vi "LSMcontroller_v56_from here for labview64bit.vi"() -> ()   [LabVIEW 2015] (continued)
                                tunnel: w3219 -> [_ w3224]
                                frame False {
                                }
                                frame True {
                                n918 = Quotient & Remainder(x=w3224, y=u32 2 ("min phot")) -> (floor(x/y)=w3223:u32)  [unwired: 1 out]
                                n919 = Max & Min(x=w3223, y=u32 5) -> (max(x,y)=w3222:u32)  [unwired: 1 out]
                                n920 = local write "min phot"(w3222) -> ()
                                }
                                }
                                n921 = To Double Precision Float(number=w3209) -> (double precision float=w3210:dbl)
                                n922 = local write "img_CH1"(w3211) -> ()
                                n923 = property on="img_CH1" class="IntGraph (strict)"("ZScale.Maximum"=w3210) -> ()  [unwired: 2 in, 2 out]
                                }
                                }
                                }
                                frame #4 {
                                w3228 = u16 1 items=["Stream to disk", "Post process", "real time process"] ("Ring")
                                n924 = local read "T3R Data processing"() -> (w3227:u16)
                                n925 = Equal?(x=w3227, y=w3228) -> (x = y?=w3226:bool)
                                n926 = case shown="False" w3226 {
                                frame False {
                                # "intensity"
                                n927 = local read "Current Average"() -> (w3233:sgl)
                                n928 = local read "image2list"() -> (w3229:u16)
                                n929 = local read "image1list"() -> (w3230:u16)
                                n930 = call "dattoimage.vi"("image2list"=w3229, "Current Average"=w3233, "image1list"=w3230) -> ("image 1 array out"=w3232:sgl[][])  [unwired: 1 out]
                                n931 = Transpose 2D Array(2D array=w3232) -> (transposed array=w3231:sgl[][])
                                n932 = local write "img_CH2"(w3231) -> ()
                                }
                                frame True {
                                }
                                }
                                }
                                }
                              }
                              frame Enabled {
                              }
                            }
                          }
                        }
                        n933 = local write "64bit disabled"(TRUE ("64bit disabled")) -> ()
                      }
                      frame #9 {
                        n934 = call "2pparameters.vi"("command"="get") -> ("params out"=w3236:T12)  [unwired: 1 in]
                        n935 = Unbundle By Name(w3236) -> ("auto OD"=w3235:bool)
                        n936 = case shown="True" w3235 {
                          frame False {
                          }
                          frame True {
                            n937 = call "configuration.vi"("command"="get") -> ("config out"=w3239:T13)  [unwired: 2 in, 1 out]
                            n938 = call "2pparameters.vi"("command"="get") -> ("params out"=w3242:T12)  [unwired: 1 in]
                            n939 = Unbundle By Name(w3239) -> ("image OD"=w3237:u16)
                            n940 = Unbundle By Name(w3242) -> ("ODfilt"=w3238:u16)
                            n941 = call "filterwheelcontrol_nothorlabslib.vi"("Current OD filt"=w3237, "New ODfilt"=w3238) -> ()  [unwired: 1 in]
                          }
                        }
                        n942 = call "reset AO_DO_v3.vi"() -> ()  [unwired: 12 in]
                      }
                      frame #10 {
                        n943 = stacked-sequence {
                          tunnel: w3256 -> [w3259 _ _ _ _ _]
                          tunnel: w3255 -> [w3258 _ _ _ _ _]
                          tunnel: w3254 -> [w3257 _ _ _ _ _]
                          tunnel: w3253 -> [_ w3308 _ _ _ _]
                          tunnel: w3252 -> [_ w3307 w3362 w3459 _ _]
                          tunnel: w3251 -> [_ w3306 w3361 w3458 _ _]
                          tunnel: w3250 -> [_ _ w3360 _ _ _]
                          tunnel: w3249 -> [_ _ w3359 _ _ _]
                          tunnel: w3248 -> [_ _ _ w3457 _ _]
                          tunnel: w3247 -> [_ _ _ w3456 _ _]
                          tunnel: w3246 -> [_ _ w3357 _ _ _]
                          tunnel: w3245 -> [_ _ w3356 _ _ _]
                          tunnel: w3244 -> [_ _ _ w3454 _ _]
                          tunnel: w3243 -> [_ _ _ w3453 _ _]
                          frame #0 {
                            n944 = case shown="False" w3259 {
                              tunnel: w3258 -> [_ w3281]
                              tunnel: w3257 -> [_ w3280]
                              frame True {
                                n945 = stacked-sequence {
                                seq-local: [w3260 _ _] -> [_ w3272 w3277]
                                frame #0 {
                                n946 = call "configuration.vi"("command"="get") -> ("config out"=w3266:T13)  [unwired: 2 in, 1 out]
                                n947 = Unbundle By Name(w3266) -> ("Voltage to Xgalvo"=w3263:i32)
                                n948 = call "2pparameters.vi"("command"="get") -> ("params out"=w3264:T12)  [unwired: 1 in]
                                n949 = in-place {
                                in-place-border: w3263 -> [w3271]
                                in-place-border: [w3268] -> w3260
                                n950 = in-place-cluster #9(w3264) -> ("aAO"=w3270:u32[])
                                n951 = call "remove channel from active arrayv2.vi"("line array in"=w3270, "line to remove"=w3271) -> ("line array out"=w3269:u32[], "index"=w3268:i32)  [unwired: 1 out]
                                n952 = in-place-cluster #9("aAO"=w3269) -> (w3261:T12)
                                }
                                n953 = call "2pparameters.vi"("Params in"=w3261, "command"="set") -> ()  [unwired: 1 out]
                                }
                                frame #1 {
                                n954 = call "waveformparamsv2.vi"("command"="rem AO", "index"=w3272) -> ()  [unwired: 3 in, 3 out]
                                }
                                frame #2 {
                                n955 = call "waveformsAObuffer.vi"("command"="get") -> ("AO wf out"=w3278:waveform(dbl)[])  [unwired: 1 in]
                                n956 = Delete From Array(array=w3278, length=1, index=w3277) -> (array with subset deleted=w3274:waveform(dbl)[])  [unwired: 1 out]
                                n957 = call "waveformsAObuffer.vi"("AO wf in"=w3274, "command"="set") -> ()  [unwired: 1 out]
                                }
                                }
                              }
                              frame False {
                                n958 = stacked-sequence {
                                seq-local: [w3282 _ _] -> [_ w3290 w3301]
                                tunnel: w3281 -> [_ w3289 _]
                                tunnel: w3280 -> [_ _ w3300]
                                frame #0 {
                                n959 = call "configuration.vi"("command"="get") -> ("config out"=w3287:T13)  [unwired: 2 in, 1 out]
                                n960 = Unbundle By Name(w3287) -> ("Voltage to Xgalvo"=w3283:i32)
                                n961 = call "2pparameters.vi"("command"="get") -> ("params out"=w3286:T12)  [unwired: 1 in]
                                n962 = Unbundle By Name(w3286) -> ("aAO"=w3284:u32[])
                                n963 = Search 1D Array(1D array=w3284, element=w3283) -> (index of element=w3282:i32)  [unwired: 1 in]
                                }
                                frame #1 {
                                n964 = call "waveformparamsv2.vi"("command"="get") -> ("Params out"=w3293:T16)  [unwired: 4 in, 2 out]
                                n965 = in-place {
                                in-place-border: w3290 -> [w3297]
                                in-place-border: w3289 -> [w3296]
                                n966 = in-place-cluster #10(w3293) -> ("AO parameters"=w3298:T17)
                                n967 = in-place {
                                in-place-border: w3296 -> [w3299]
                                n968 = in-place-array #11(w3298, w3297) -> ()  [unwired: 1 out]
                                n969 = in-place-array #11(w3299) -> (w3295:T17)  [unwired: 1 out]
                                }
                                n970 = in-place-cluster #10("AO parameters"=w3295) -> (w3291:T16)
                                }
                                n971 = call "waveformparamsv2.vi"("command"="set", "Params in"=w3291) -> ()  [unwired: 3 in, 3 out]
                                }
                                frame #2 {
                                n972 = call "waveformsAObuffer.vi"("command"="get") -> ("AO wf out"=w3304:waveform(dbl)[])  [unwired: 1 in]
                                n973 = Replace Array Subset(array=w3304, new element=w3300, index=w3301) -> (w3302:waveform(dbl)[])
                                n974 = call "waveformsAObuffer.vi"("AO wf in"=w3302, "command"="set") -> ()  [unwired: 1 out]
                                }
                                }
                              }
                            }
                          }
                          frame #1 {
                            n975 = case shown="True" w3308 {
                              tunnel: w3307 -> [_ w3330]
                              tunnel: w3306 -> [_ w3329]
                              frame True {
                                n976 = stacked-sequence {
                                seq-local: [w3309 _ _] -> [_ w3321 w3326]
                                frame #0 {
                                n977 = call "configuration.vi"("command"="get") -> ("config out"=w3315:T13)  [unwired: 2 in, 1 out]
                                n978 = Unbundle By Name(w3315) -> ("Voltage to Ygalvo"=w3312:i32)
                                n979 = call "2pparameters.vi"("command"="get") -> ("params out"=w3313:T12)  [unwired: 1 in]
                                n980 = in-place {
                                in-place-border: w3312 -> [w3320]
                                in-place-border: [w3317] -> w3309
                                n981 = in-place-cluster #12(w3313) -> ("aAO"=w3319:u32[])
                                n982 = call "remove channel from active arrayv2.vi"("line array in"=w3319, "line to remove"=w3320) -> ("line array out"=w3318:u32[], "index"=w3317:i32)  [unwired: 1 out]
                                n983 = in-place-cluster #12("aAO"=w3318) -> (w3310:T12)
                                }
                                n984 = call "2pparameters.vi"("Params in"=w3310, "command"="set") -> ()  [unwired: 1 out]
                                }
                                frame #1 {
                                n985 = call "waveformparamsv2.vi"("command"="rem AO", "index"=w3321) -> ()  [unwired: 3 in, 3 out]
                                }
                                frame #2 {
                                n986 = call "waveformsAObuffer.vi"("command"="get") -> ("AO wf out"=w3327:waveform(dbl)[])  [unwired: 1 in]
                                n987 = Delete From Array(array=w3327, length=1, index=w3326) -> (array with subset deleted=w3323:waveform(dbl)[])  [unwired: 1 out]
                                n988 = call "waveformsAObuffer.vi"("AO wf in"=w3323, "command"="set") -> ()  [unwired: 1 out]
                                }
                                }
                              }
                              frame False {
                                n989 = stacked-sequence {
                                seq-local: [w3331 _ _] -> [_ w3339 w3350]
                                tunnel: w3330 -> [_ w3338 _]
                                tunnel: w3329 -> [_ _ w3349]
                                frame #0 {
                                n990 = call "configuration.vi"("command"="get") -> ("config out"=w3336:T13)  [unwired: 2 in, 1 out]
                                n991 = Unbundle By Name(w3336) -> ("Voltage to Ygalvo"=w3332:i32)
                                n992 = call "2pparameters.vi"("command"="get") -> ("params out"=w3335:T12)  [unwired: 1 in]
                                n993 = Unbundle By Name(w3335) -> ("aAO"=w3333:u32[])
                                n994 = Search 1D Array(1D array=w3333, element=w3332) -> (index of element=w3331:i32)  [unwired: 1 in]
                                }
                                frame #1 {
                                n995 = call "waveformparamsv2.vi"("command"="get") -> ("Params out"=w3342:T16)  [unwired: 4 in, 2 out]
                                n996 = in-place {
                                in-place-border: w3339 -> [w3346]
                                in-place-border: w3338 -> [w3345]
                                n997 = in-place-cluster #13(w3342) -> ("AO parameters"=w3347:T17)
                                n998 = in-place {
                                in-place-border: w3345 -> [w3348]
                                n999 = in-place-array #14(w3347, w3346) -> ()  [unwired: 1 out]
                                n1000 = in-place-array #14(w3348) -> (w3344:T17)  [unwired: 1 out]
                                }
                                n1001 = in-place-cluster #13("AO parameters"=w3344) -> (w3340:T16)
                                }
                                n1002 = call "waveformparamsv2.vi"("command"="set", "Params in"=w3340) -> ()  [unwired: 3 in, 3 out]
                                }
                                frame #2 {
                                n1003 = call "waveformsAObuffer.vi"("command"="get") -> ("AO wf out"=w3353:waveform(dbl)[])  [unwired: 1 in]
                                n1004 = Replace Array Subset(array=w3353, new element=w3349, index=w3350) -> (w3351:waveform(dbl)[])
                                n1005 = call "waveformsAObuffer.vi"("AO wf in"=w3351, "command"="set") -> ()  [unwired: 1 out]
                                }
                                }
                              }
                            }
                          }
                          frame #2 {
                            n1006 = Build Array(w3357, w3356) -> (w3355:bool[])
                            n1007 = Boolean Array To Number(Boolean array=w3355) -> (number=w3358:u32)
                            n1008 = case shown="0" w3358 {
                              tunnel: w3362 -> [_ _ w3405]
                              tunnel: w3361 -> [_ _ w3404]
                              tunnel: w3360 -> [_ w3384 w3402]
                              tunnel: w3359 -> [_ w3383 w3403]
                              frame 1, Default {
                                n1009 = stacked-sequence {
                                seq-local: [w3363 _ _] -> [_ w3375 w3380]
                                frame #0 {
                                n1010 = call "configuration.vi"("command"="get") -> ("config out"=w3369:T13)  [unwired: 2 in, 1 out]
                                n1011 = Unbundle By Name(w3369) -> ("2P shutter"=w3366:i32)
                                n1012 = call "2pparameters.vi"("command"="get") -> ("params out"=w3367:T12)  [unwired: 1 in]
                                n1013 = in-place {
                                in-place-border: w3366 -> [w3374]
                                in-place-border: [w3371] -> w3363
                                n1014 = in-place-cluster #15(w3367) -> ("aDO"=w3373:u32[])
                                n1015 = call "remove channel from active arrayv2.vi"("line array in"=w3373, "line to remove"=w3374) -> ("line array out"=w3372:u32[], "index"=w3371:i32)  [unwired: 1 out]
                                n1016 = in-place-cluster #15("aDO"=w3372) -> (w3364:T12)
                                }
                                n1017 = call "2pparameters.vi"("Params in"=w3364, "command"="set") -> ()  [unwired: 1 out]
                                }
                                frame #1 {
                                n1018 = call "waveformparamsv2.vi"("command"="rem DO", "index"=w3375) -> ()  [unwired: 3 in, 3 out]
                                }
                                frame #2 {
                                n1019 = call "waveformsDObuffer.vi"("command"="get") -> ("DO wf out"=w3381:digitalwaveform[])  [unwired: 1 in]
                                n1020 = Delete From Array(array=w3381, length=1, index=w3380) -> (array with subset deleted=w3377:digitalwaveform[])  [unwired: 1 out]
                                n1021 = call "waveformsDObuffer.vi"("DO wf in"=w3377, "command"="set") -> ()  [unwired: 1 out]
                                }
                                }
                              }
                              frame 2 {
                                n1022 = stacked-sequence {
                                tunnel: w3384 -> [_ w3395 _]
                                tunnel: w3383 -> [_ _ w3399]
                                frame #0 {
                                n1023 = call "configuration.vi"("command"="get") -> ("config out"=w3386:T13)  [unwired: 2 in, 1 out]
                                n1024 = call "2pparameters.vi"("command"="get") -> ("params out"=w3390:T12)  [unwired: 1 in]
                                n1025 = Unbundle By Name(w3386) -> ("2P shutter"=w3385:i32)
                                n1026 = in-place {
                                in-place-border: w3385 -> [w3394]
                                n1027 = in-place-cluster #16(w3390) -> ("aDO"=w3393:u32[])
                                n1028 = call "add channel to active arrayv2.vi"("line array in"=w3393, "line to add"=w3394) -> ("line array out"=w3392:u32[])  [unwired: 2 out]
                                n1029 = in-place-cluster #16("aDO"=w3392) -> (w3388:T12)
                                }
                                n1030 = call "2pparameters.vi"("Params in"=w3388, "command"="set") -> ()  [unwired: 1 out]
                                }
                                frame #1 {
                                n1031 = call "waveformparamsv2.vi"("command"="add DO", "add DO"=w3395) -> ()  [unwired: 3 in, 3 out]
                                }
                                frame #2 {
                                n1032 = call "waveformsDObuffer.vi"("command"="get") -> ("DO wf out"=w3400:digitalwaveform[])  [unwired: 1 in]
                                n1033 = Build Array (concatenate)(w3400, w3399) -> (w3398:digitalwaveform[])
                                n1034 = call "waveformsDObuffer.vi"("DO wf in"=w3398, "command"="set") -> ()  [unwired: 1 out]
                                }
                                }
                              }
                              frame 0 {
                                n1035 = stacked-sequence {
                                seq-local: [w3406 _ _] -> [_ w3414 w3436]
                                tunnel: w3405 -> [_ _ _]
                                tunnel: w3404 -> [_ _ _]
                                tunnel: w3403 -> [_ _ w3435]
                                tunnel: w3402 -> [_ w3413 _]
                                frame #0 {
                                n1036 = call "configuration.vi"("command"="get") -> ("config out"=w3411:T13)  [unwired: 2 in, 1 out]
                                n1037 = call "2pparameters.vi"("command"="get") -> ("params out"=w3410:T12)  [unwired: 1 in]
                                n1038 = Unbundle By Name(w3411) -> ("2P shutter"=w3407:i32)
                                n1039 = Unbundle By Name(w3410) -> ("aDO"=w3408:u32[])
                                n1040 = Search 1D Array(1D array=w3408, element=w3407) -> (index of element=w3406:i32)  [unwired: 1 in]
                                }
                                frame #1 {
                                n1041 = call "2pparameters.vi"("command"="get") -> ("params out"=w3417:T12)  [unwired: 1 in]
                                n1042 = Unbundle By Name(w3417) -> ("wavdet"=w3415:bool, "autoshutter"=w3416:bool)
                                n1043 = case shown="True" w3416 {
                                tunnel: w3414 -> [_ w3421]
                                tunnel: w3415 -> [_ w3420]
                                tunnel: w3413 -> [_ w3419]
                                frame False {
                                }
                                frame True {
                                n1044 = case shown="False" w3420 {
                                tunnel: w3421 -> [w3425 _]
                                tunnel: w3419 -> [w3423 _]
                                frame False {
                                n1045 = Index Array(array=w3423, index=0) -> (element=w3422:T20)
                                n1046 = call "waveformparamsv2.vi"("command"="get") -> ("Params out"=w3428:T16)  [unwired: 4 in, 2 out]
                                n1047 = in-place {
                                in-place-border: w3425 -> [w3432]
                                in-place-border: w3422 -> [w3430]
                                n1048 = in-place-cluster #17(w3428) -> ("DO parameters"=w3433:T19)
                                n1049 = in-place {
                                in-place-border: w3430 -> [w3434]
                                n1050 = in-place-array #18(w3433, w3432) -> ()  [unwired: 1 out]
                                n1051 = in-place-array #18(w3434) -> (w3431:T19)  [unwired: 1 out]
                                }
                                n1052 = in-place-cluster #17("DO parameters"=w3431) -> (w3426:T16)
                                }
                                n1053 = call "waveformparamsv2.vi"("command"="set", "Params in"=w3426) -> ()  [unwired: 3 in, 3 out]
                                }
                                frame True {
                                }
                                }
                                }
                                }
                                }
                                frame #2 {
                                n1054 = call "2pparameters.vi"("command"="get") -> ("params out"=w3439:T12)  [unwired: 1 in]
                                n1055 = Unbundle By Name(w3439) -> ("wavdet"=w3437:bool, "autoshutter"=w3438:bool)
                                n1056 = case shown="True" w3438 {
                                tunnel: w3436 -> [_ w3443]
                                tunnel: w3437 -> [_ w3442]
                                tunnel: w3435 -> [_ w3441]
                                frame False {
                                }
                                frame True {
                                n1057 = case shown="False" w3442 {
                                tunnel: w3443 -> [w3447 _]
                                tunnel: w3441 -> [w3446 _]
                                frame False {
                                n1058 = Index Array(array=w3446, index=0) -> (element=w3444:digitalwaveform)
                                n1059 = call "waveformsDObuffer.vi"("command"="get") -> ("DO wf out"=w3449:digitalwaveform[])  [unwired: 1 in]
                                n1060 = Replace Array Subset(array=w3449, new element=w3444, index=w3447) -> (w3451:digitalwaveform[])
                                n1061 = call "waveformsDObuffer.vi"("DO wf in"=w3451, "command"="set") -> ()  [unwired: 1 out]
                                }
                                frame True {
                                }
                                }
                                }
                                }
                                }
                                }
                              }
                            }
                          }
                          frame #3 {
                            n1062 = Build Array(w3454, w3453) -> (w3455:bool[])
                            n1063 = Boolean Array To Number(Boolean array=w3455) -> (number=w3452:u32)
                            n1064 = case shown="0" w3452 {
                              tunnel: w3459 -> [_ _ w3502]
                              tunnel: w3458 -> [_ _ w3501]
                              tunnel: w3457 -> [_ w3481 w3499]
                              tunnel: w3456 -> [_ w3480 w3500]
                              frame 1, Default {
                                n1065 = stacked-sequence {
                                seq-local: [w3460 _ _] -> [_ w3472 w3477]
                                frame #0 {
                                n1066 = call "configuration.vi"("command"="get") -> ("config out"=w3466:T13)  [unwired: 2 in, 1 out]
                                n1067 = Unbundle By Name(w3466) -> ("LT timestamp"=w3463:u32)
                                n1068 = call "2pparameters.vi"("command"="get") -> ("params out"=w3464:T12)  [unwired: 1 in]
                                n1069 = in-place {
                                in-place-border: w3463 -> [w3471]
                                in-place-border: [w3468] -> w3460
                                n1070 = in-place-cluster #19(w3464) -> ("aDO"=w3470:u32[])
                                n1071 = call "remove channel from active arrayv2.vi"("line array in"=w3470, "line to remove"=w3471) -> ("line array out"=w3469:u32[], "index"=w3468:i32)  [unwired: 1 out]
                                n1072 = in-place-cluster #19("aDO"=w3469) -> (w3461:T12)
                                }
                                n1073 = call "2pparameters.vi"("Params in"=w3461, "command"="set") -> ()  [unwired: 1 out]
                                }
                                frame #1 {
                                n1074 = call "waveformparamsv2.vi"("command"="rem DO", "index"=w3472) -> ()  [unwired: 3 in, 3 out]
                                }
                                frame #2 {
                                n1075 = call "waveformsDObuffer.vi"("command"="get") -> ("DO wf out"=w3478:digitalwaveform[])  [unwired: 1 in]
                                n1076 = Delete From Array(array=w3478, length=1, index=w3477) -> (array with subset deleted=w3474:digitalwaveform[])  [unwired: 1 out]
                                n1077 = call "waveformsDObuffer.vi"("DO wf in"=w3474, "command"="set") -> ()  [unwired: 1 out]
                                }
                                }
                              }
                              frame 2 {
                                n1078 = stacked-sequence {
                                tunnel: w3481 -> [_ _ w3494]
                                tunnel: w3480 -> [_ w3492 _]
                                frame #0 {
                                n1079 = call "configuration.vi"("command"="get") -> ("config out"=w3483:T13)  [unwired: 2 in, 1 out]
                                n1080 = Unbundle By Name(w3483) -> ("LT timestamp"=w3482:u32)
                                n1081 = call "2pparameters.vi"("command"="get") -> ("params out"=w3487:T12)  [unwired: 1 in]
                                n1082 = in-place {
                                in-place-border: w3482 -> [w3491]
                                n1083 = in-place-cluster #20(w3487) -> ("aDO"=w3490:u32[])
                                n1084 = call "add channel to active arrayv2.vi"("line array in"=w3490, "line to add"=w3491) -> ("line array out"=w3489:u32[])  [unwired: 2 out]
                                n1085 = in-place-cluster #20("aDO"=w3489) -> (w3485:T12)
                                }
                                n1086 = call "2pparameters.vi"("Params in"=w3485, "command"="set") -> ()  [unwired: 1 out]
                                }
                                frame #1 {
                                n1087 = call "waveformparamsv2.vi"("command"="add DO", "add DO"=w3492) -> ()  [unwired: 3 in, 3 out]
                                }
                                frame #2 {
                                n1088 = call "waveformsDObuffer.vi"("command"="get") -> ("DO wf out"=w3497:digitalwaveform[])  [unwired: 1 in]
                                n1089 = Build Array (concatenate)(w3497, w3494) -> (w3496:digitalwaveform[])
                                n1090 = call "waveformsDObuffer.vi"("DO wf in"=w3496, "command"="set") -> ()  [unwired: 1 out]
                                }
                                }
                              }
                              frame 0 {
                                n1091 = stacked-sequence {
                                seq-local: [w3503 _ _] -> [_ w3513 w3530]
                                tunnel: w3502 -> [_ _ _]
                                tunnel: w3501 -> [_ _ _]
                                tunnel: w3500 -> [_ w3510 _]
                                tunnel: w3499 -> [_ _ w3529]
                                frame #0 {
                                n1092 = call "configuration.vi"("command"="get") -> ("config out"=w3508:T13)  [unwired: 2 in, 1 out]
                                n1093 = Unbundle By Name(w3508) -> ("LT timestamp"=w3504:u32)
                                n1094 = call "2pparameters.vi"("command"="get") -> ("params out"=w3507:T12)  [unwired: 1 in]
                                n1095 = Unbundle By Name(w3507) -> ("aDO"=w3505:u32[])
                                n1096 = Search 1D Array(1D array=w3505, element=w3504) -> (index of element=w3503:i32)  [unwired: 1 in]
                                }
                                frame #1 {
                                n1097 = local read "Measurement"() -> (w3512:T5)
                                n1098 = To Unsigned Long Integer(number=w3512) -> (unsigned 32bit integer=w3511:u32)
                                n1099 = case shown="5..7" w3511 {
                                tunnel: w3513 -> [_ w3517]
                                tunnel: w3510 -> [_ w3514]
                                frame 0..4, Default {
                                }
                                frame 5..7 {
                                n1100 = Index Array(array=w3514, index=0) -> (element=w3515:T20)
                                n1101 = call "waveformparamsv2.vi"("command"="get") -> ("Params out"=w3520:T16)  [unwired: 4 in, 2 out]
                                n1102 = in-place {
                                in-place-border: w3517 -> [w3524]
                                in-place-border: w3515 -> [w3522]
                                n1103 = in-place-cluster #21(w3520) -> ("DO parameters"=w3525:T19)
                                n1104 = in-place {
                                in-place-border: w3522 -> [w3526]
                                n1105 = in-place-array #22(w3525, w3524) -> ()  [unwired: 1 out]
                                n1106 = in-place-array #22(w3526) -> (w3523:T19)  [unwired: 1 out]
                                }
                                n1107 = in-place-cluster #21("DO parameters"=w3523) -> (w3518:T16)
                                }
                                n1108 = call "waveformparamsv2.vi"("command"="set", "Params in"=w3518) -> ()  [unwired: 3 in, 3 out]
                                }
                                }
                                }
                                frame #2 {
                                n1109 = local read "Measurement"() -> (w3528:T5)
                                n1110 = To Unsigned Long Integer(number=w3528) -> (unsigned 32bit integer=w3527:u32)
                                n1111 = case shown="5..7" w3527 {
                                tunnel: w3530 -> [_ w3534]
                                tunnel: w3529 -> [_ w3532]
                                frame 0..4, Default {
                                }
                                frame 5..7 {
                                n1112 = Index Array(array=w3532, index=0) -> (element=w3531:digitalwaveform)
                                n1113 = call "waveformsDObuffer.vi"("command"="get") -> ("DO wf out"=w3536:digitalwaveform[])  [unwired: 1 in]
                                n1114 = Replace Array Subset(array=w3536, new element=w3531, index=w3534) -> (w3538:digitalwaveform[])
                                n1115 = call "waveformsDObuffer.vi"("DO wf in"=w3538, "command"="set") -> ()  [unwired: 1 out]
                                }
                                }
                                }
                                }
                              }
                            }
                          }
                          frame #4 {
                            n1116 = call "Used AO lines.vi"() -> ("used AO names"=w3541:string[], "used AO lines"=w3539:tag[])  [unwired: 2 in]
                            n1117 = control-ref of="Analog Lines Plot"() -> (w3540:refnum<vi>)
                            n1118 = control-ref of="Digital Lines Plot"() -> (w3542:refnum<vi>)
                            n1119 = call "Used DO lines.vi"() -> ("used DO names"=w3543:string[], "used DO lines"=w3544:tag[])  [unwired: 2 in]
                            n1120 = local write "Analog Used Lines"(w3539) -> ()
                            n1121 = local write "Analog Used Names"(w3541) -> ()
                            n1122 = local write "Digital Used Lines"(w3544) -> ()
                            n1123 = local write "Digital Used Names"(w3543) -> ()
                            n1124 = call "prepDOWaveplot.vi"("DigitalGraph in"=w3542, "used DO names"=w3543) -> ()  [unwired: 1 in]
                            n1125 = call "prepAOWaveplot.vi"("WaveformGraph in"=w3540, "Analog Used Names"=w3541) -> ()  [unwired: 1 in]
                          }
                          frame #5 {
                            n1126 = local read "Meastab"() -> (w3559:enum32{"X-Y Image", "Linescan", "Timetrace"})
                            n1127 = property on="refwf" class="Ring (strict)"() -> ("RingText.Text"=w3556:string)  [unwired: 2 in, 2 out]
                            n1128 = case shown="\"Timetrace\"" w3559 {
                              tunnel: [w3561 w3562] -> w3560
                              frame "X-Y Image", Default {
                                n1129 = local read "Sampling rate"() -> (w3561:dbl)
                              }
                              frame "Timetrace" {
                                n1130 = local read "srateAODOtt"() -> (w3562:dbl)
                              }
                            }
                            n1131 = call "waveformsAObuffer.vi"("command"="get") -> ("AO wf out"=w3547:waveform(dbl)[])  [unwired: 1 in]
                            n1132 = local read "wavdet"() -> (w3557:bool)
                            n1133 = call "waveformsDObuffer.vi"("command"="get") -> ("DO wf out"=w3551:digitalwaveform[])  [unwired: 1 in]
                            n1134 = call "correctwaveformsizetemp.vi"("new sampling frequency (Hz)"=w3560, "start"=FALSE, "reference waveforms to"=w3556, "Analog waveforms in"=w3547, "stop"=TRUE, "Digital waveforms in"=w3551) -> ("analog wf out"=w3553:waveform(dbl)[], "Digital wf out"=w3555:digitalwaveform[], "measpoints"=w3558:i32)
                            n1135 = local write "Analog Lines Plot"(w3553) -> ()
                            n1136 = call "GetNumCamFramesv2.vi"("Digital Waveform Graph"=w3555) -> ("Numeric"=w3554:i32)  [unwired: 10 in]
                            n1137 = local write "Digital Lines Plot"(w3555) -> ()
                            n1138 = call "waveformsDObuffer.vi"("DO wf in"=w3555, "command"="set") -> ()  [unwired: 1 out]
                            n1139 = call "waveformsAObuffer.vi"("AO wf in"=w3553, "command"="set") -> ()  [unwired: 1 out]
                            n1140 = local write "Total Camera Frames"(w3554) -> ()
                            n1141 = case shown="True" w3557 {
                              tunnel: w3558 -> [_ w3563]
                              frame False {
                              }
                              frame True {
                                n1142 = local write "# of frames"(w3563) -> ()
                              }
                            }
                          }
                        }
                        n1143 = call "stoperaseCI.vi"() -> ()  [unwired: 12 in]
                        n1144 = call "stoperaseDO_img.vi"() -> ()  [unwired: 12 in]
                        n1145 = call "stoperaseAO_img.vi"() -> ()  [unwired: 12 in]
                        n1146 = call "stoperaseAI_img.vi"() -> ()  [unwired: 12 in]
                      }
                      frame #11 {
                        w3571 = FALSE ("Value (Signaling)")
                        n1147 = local read "save\ndata"() -> (w3564:bool)
                        n1148 = local read "save\ndata"() -> (w3565:bool)
                        n1149 = property on="Stop" class="Bool (strict)"("Visible"=FALSE, "DisabledEnum"=T8."Disabled" ("Disabled")) -> ()  [unwired: 2 in, 2 out]
                        n1150 = case shown="True" w3564 {
                          frame False {
                          }
                          frame True {
                            n1151 = call "closetiffs.vi"() -> ()  [unwired: 12 in]
                          }
                        }
                        n1152 = case shown="True" w3565 {
                          tunnel: w3566 -> [_ w3572]
                          frame False {
                          }
                          frame True {
                            n1153 = local read "filename prefix"() -> (w3574:string)
                            n1154 = local read "data dir"() -> (w3573:path)
                            n1155 = call "savetimestamps.vi"("timestamp"=w3572, "filename prefix in"=w3574, "data dir in"=w3573) -> ()  [unwired: 1 in]
                            n1156 = call "saveparams.vi"("filename prefix in"=w3574, "data dir in"=w3573) -> ()  [unwired: 2 in]
                          }
                        }
                        n1157 = property on="Start" class="Bool (strict)"("Visible"=TRUE, "DisabledEnum"=T8."Enabled" ("Disabled")) -> ()  [unwired: 2 in, 2 out]
                        n1158 = property on="Start" class="Bool (strict)"("Val(Sgnl)"=w3571) -> ()  [unwired: 2 in, 2 out]
                        n1159 = property on="Stop" class="Bool (strict)"("Val(Sgnl)"=w3571) -> ()  [unwired: 2 in, 2 out]
                      }
                      frame #12 {
                        w3578 = T23 2 items=["no dialog", "OK message", "continue or stop message", "OK message + warnings", "continue/stop + warnings"] ("type of dialog (OK msg:1)")
                        n1160 = call "displayerrors.vi"() -> ("error IO"=w3577:errorcluster)
                        n1161 = call <vilib>:"General Error Handler.vi"("type of dialog (OK msg:1)"=w3578, "error in (no error)"=w3577) -> ("error out"=w3576:errorcluster)  [unwired: 9 in, 4 out]
                        n1162 = call <vilib>:"Clear Errors.vi"("error in (no error)"=w3576) -> ("error out"=w3575:errorcluster)  [unwired: 5 in, 1 out]
                        n1163 = call "seterrors.vi"("error IO"=w3575) -> ()
                      }
                    }
                  }
                  frame "X-Y-Z-t movie" {
                    n1164 = call "2pparameters.vi"("command"="get") -> ("params out"=w3581:T12)  [unwired: 1 in]
                    n1165 = Bundle By Name(cluster=w3581, "type"="X-Y-Z-t movie") -> (w3579:T12)
                    n1166 = call "2pparameters.vi"("Params in"=w3579, "command"="set") -> ()  [unwired: 1 out]
                  }
                  frame "linescan" {
                    n1167 = call "2pparameters.vi"("command"="get") -> ("params out"=w3586:T12)  [unwired: 1 in]
                    n1168 = Bundle By Name(cluster=w3586, "type"="linescan") -> (w3588:T12)
                    n1169 = call "2pparameters.vi"("Params in"=w3588, "command"="set") -> ()  [unwired: 1 out]
                  }
                  frame "Timetrace", "Lifetime (contour)" {
                    n1170 = local read "ttt"() -> (w3589:T4)
                    n1171 = case shown="\"Resonant Ellipse\", \"freeform contour\"" w3589 {
                      frame "Point", Default {
                        n1172 = stacked-sequence {
                          seq-local: [w3590 _ _ _ _ _ _ _ _] -> [_ _ w3723 _ _ _ _ _ w3781]
                          frame #0 {
                            n1173 = Get Date/Time In Seconds() -> (seconds since 1Jan1904=w3591:timestamp)
                            n1174 = call "createdatafolder.vi"("timestamp in"=w3591) -> ("current data path"=w3592:path, "timestamp out"=w3590:timestamp)
                            n1175 = stacked-sequence {
                              frame #0 {
                                n1176 = call "2pparameters.vi"("command"="get") -> ("params out"=w3607:T12)  [unwired: 1 in]
                                n1177 = Bundle By Name(cluster=w3607, "type"="Timetrace") -> (w3605:T12)
                                n1178 = call "2pparameters.vi"("command"="get") -> ("params out"=w3596:T12)  [unwired: 1 in]
                                n1179 = local write "graphtab"(T6."timetrace" ("graphtab")) -> ()
                                n1180 = Unbundle By Name(w3596) -> ("Vx-min Img"=w3598:dbl, "VX-max Img"=w3597:dbl, "Vy-min Img"=w3600:dbl, "Vy-max Img"=w3599:dbl, "Angle Img"=w3601:dbl)
                                n1181 = property on="Stop" class="Bool (strict)"("Visible"=TRUE, "DisabledEnum"=T8."Enabled" ("Disabled")) -> ()  [unwired: 2 in, 2 out]
                                n1182 = property on="Start" class="Bool (strict)"("Visible"=FALSE, "DisabledEnum"=T8."Disabled and Grayed Out" ("Disabled")) -> ()  [unwired: 2 in, 2 out]
                                n1183 = local read "Vy-ref"() -> (w3603:dbl)
                                n1184 = local read "Vx-ref"() -> (w3602:dbl)
                                n1185 = call "2pparameters.vi"("Params in"=w3605, "command"="set") -> ()  [unwired: 1 out]
                                n1186 = script code="Xic=(ximax+ximin)./2;\nYic=(yimax+yimin)./2;\nx=x-Xic;\ny=y-Yic;\nxout=x.*cos(pi/180.*phi)+y.*sin(pi./180.*phi)+Xic;\nyout=-x.*sin(pi./180.*phi)+y.*cos(pi./180.*phi)+Yic;"("ximax"=w3597, "ximin"=w3598, "yimax"=w3599, "yimin"=w3600, "phi"=w3601, "x"=w3602, "y"=w3603) -> ("xout"=w3594:dbl, "yout"=w3593:dbl)  [unwired: 1 in, 1 out]
                                n1187 = call "setposition.vi"("Vy"=w3593, "Vx"=w3594) -> ()  [unwired: 1 in]
                              }
                              frame #1 {
                                n1188 = call "2pparameters.vi"("command"="get") -> ("params out"=w3616:T12)  [unwired: 1 in]
                                n1189 = Unbundle By Name(w3616) -> ("autoshutter"=w3617:bool, "auto OD"=w3614:bool)
                                n1190 = case shown="True" w3614 {
                                frame False {
                                }
                                frame True {
                                n1191 = call "configuration.vi"("command"="get") -> ("config out"=w3620:T13)  [unwired: 2 in, 1 out]
                                n1192 = Unbundle By Name(w3620) -> ("point OD"=w3621:u16)
                                n1193 = local read "ODfilt"() -> (w3618:u16)
                                n1194 = call "filterwheelcontrol_nothorlabslib.vi"("Current OD filt"=w3618, "New ODfilt"=w3621) -> ()  [unwired: 1 in]
                                }
                                }
                                n1195 = case shown="True" w3617 {
                                frame False {
                                }
                                frame True {
                                n1196 = call "shuttercontrol.vi"("command"="close") -> ()  [unwired: 1 in, 1 out]
                                }
                                }
                              }
                              frame #2 {
                                n1197 = local read "refreshtime"() -> (w3626:dbl)
                                n1198 = local read "wavdet"() -> (w3642:bool)
                                n1199 = local read "finite samples"() -> (w3641:bool)
                                n1200 = local read "srateAODOtt"() -> (w3627:dbl)
                                n1201 = local read "srateAODOtt"() -> (w3643:dbl)
                                n1202 = local read "srateAODOtt"() -> (w3628:dbl)
                                n1203 = Multiply(x=w3627, y=w3626) -> (x*y=w3637:dbl)
                                n1204 = local read "# of frames"() -> (w3636:i32)
                                n1205 = Reciprocal(x=w3626) -> (1/x=w3625:dbl)
                                n1206 = To Long Integer(number=w3637) -> (32bit integer=w3635:i32)
                                n1207 = Quotient & Remainder(x=w3636, y=w3635) -> (x-y*floor(x/y)=w3632:i32, floor(x/y)=w3629:i32)
                                n1208 = local read "AI channels"() -> (w3624:i32[])
                                n1209 = local read "CI channels"() -> (w3623:i32[])
                                n1210 = Equal To 0?(x=w3632) -> (x = 0?=w3631:bool)
                                n1211 = Increment(x=w3629) -> (x+1=w3630:i32)
                                n1212 = local read "continuous"() -> (w3640:bool)
                                n1213 = local read "Vx-ref"() -> (w3634:dbl)
                                n1214 = local read "Vy-ref"() -> (w3639:dbl)
                                n1215 = Select(t=w3629, s=w3631, f=w3630) -> (s? t:f=w3633:i32)
                                n1216 = local read "avpp"() -> (w3638:i32)
                                n1217 = call "2pparameters.vi"("command"="get") -> ("params out"=w3646:T12)  [unwired: 1 in]
                                n1218 = Bundle By Name(cluster=w3646, "measpoints"=w3636, "tt_cycles"=w3633, "refreshbuffer"=w3635, "refreshrate"=w3625, "Vx-ref"=w3634, "Vy-ref"=w3639, "srate"=w3643, "finite"=w3641, "cont"=w3640, "wavdet"=w3642, "avpp"=w3638, "srateAODO"=w3628, "aAI"=w3624, "aCI"=w3623) -> (w3644:T12)
                                n1219 = call "2pparameters.vi"("Params in"=w3644, "command"="set") -> ()  [unwired: 1 out]
                              }
                              frame #3 {
                                n1220 = local read "Vholding (mV)"() -> (w3649:sgl)
                                n1221 = local read "Current Clamp"() -> (w3655:bool)
                                n1222 = local read "Voltage Clamp"() -> (w3654:bool)
                                n1223 = local read "OCgain"() -> (w3650:sgl)
                                n1224 = local read "CC_ICgain"() -> (w3653:dbl)
                                n1225 = local read "holdon"() -> (w3648:bool)
                                n1226 = call "patchparameters.vi"("command"="get") -> ("Params out"=w3657:T15)  [unwired: 1 in]
                                n1227 = Bundle By Name(cluster=w3657, "VC"=w3654, "CC"=w3655, "CC_icg (pA/mv)"=w3653, "VC_icg (mV/mV)"=10.0, "OCG (mV/pA)"=w3650, "OVG (mV/mV)"=0.1, "Vhold (mV)"=w3649, "holdon"=w3648) -> (w3656:T15)
                                n1228 = call "patchparameters.vi"("Params in"=w3656, "command"="set") -> ()  [unwired: 1 out]
                              }
                              frame #4 {
                                n1229 = local read "wavdet"() -> (w3660:bool)
                                n1230 = case shown="True" w3660 {
                                frame False {
                                }
                                frame True {
                                n1231 = stacked-sequence {
                                frame #0 {
                                n1232 = disable-structure shown="Disabled" {
                                frame Disabled {
                                w3672 = 10178 items=["Finite Samples"=10178, "Continuous Samples"=10123, "Hardware Timed Single Point"=12522] ("sample mode")
                                n1233 = call "patchparameters.vi"("command"="get") -> ("Params out"=w3665:T15)  [unwired: 1 in]
                                n1234 = Unbundle By Name(w3665) -> ("CC"=w3666:bool)
                                n1235 = case shown="True" w3666 {
                                tunnel: [w3683 w3686] -> w3663
                                frame False {
                                n1236 = call "patchparameters.vi"("command"="get") -> ("Params out"=w3684:T15)  [unwired: 1 in]
                                n1237 = Unbundle By Name(w3684) -> ("VC_icg (mV/mV)"=w3683:sgl)
                                }
                                frame True {
                                n1238 = call "patchparameters.vi"("command"="get") -> ("Params out"=w3687:T15)  [unwired: 1 in]
                                n1239 = Unbundle By Name(w3687) -> ("CC_icg (pA/mv)"=w3686:sgl)
                                }
                                }
                                n1240 = local read "refreshtime"() -> (w3662:dbl)
                                n1241 = local read "srateAODOtt"() -> (w3673:dbl)
                                n1242 = local read item#-1() -> (w3676)
                                n1243 = local read item#-1() -> (w3682)
                                n1244 = local read item#-1() -> (w3675)
                                n1245 = local read item#-1() -> (w3680)
                                n1246 = local read item#-1() -> (w3674)
                                n1247 = local read item#-1() -> (w3681)
                                n1248 = local read item#-1() -> (w3679)
                                n1249 = local read item#-1() -> (w3677)
                                n1250 = local read item#-1() -> (w3678)
                                n1251 = Reciprocal(x=w3662) -> (1/x=w3661:dbl)
                                n1252 = call "waveformparamsv2.vi"("command"="get") -> ("Params out"=w3669:T24)  [unwired: 1 in]
                                n1253 = Bundle By Name(cluster=w3669, "AO parameters"=w3674, "DO parameters"=w3675, "Duty cycle sq(%)"=w3676, "Voltage freq. sq(Hz)"=w3677, "# cycles sq"=w3678, "meastype"=T10."Manual", "sample rate"=w3673, "amp"=w3663, "sample mode"=w3672, "Min Voltage tri (mV)"=w3679, "Max voltage tri (mV)"=w3680, "Voltage freq. tri(Hz)"=w3681, "# cycles tri"=w3682, "refreshrate"=w3661) -> (w3670:T24)
                                n1254 = call "waveformparamsv2.vi"("Params in"=w3670, "command"="set") -> ()  [unwired: 1 out]
                                }
                                frame Enabled {
                                }
                                }
                                }
                                frame #1 {
                                n1255 = disable-structure shown="Disabled" {
                                frame Disabled {
                                n1256 = call "2pparameters.vi"("command"="set") -> ("params out"=w3691:T12)  [unwired: 1 in]
                                n1257 = local read item#-1() -> (w3698)
                                n1258 = local read item#-1() -> (w3697)
                                n1259 = local read item#-1() -> (w3699)
                                n1260 = Unbundle By Name(w3691) -> ("aAO"=w3690:u32[], "aDO"=w3689:u32[])
                                n1261 = call "waveformparamsv2.vi"("command"="get") -> ("Params out"=w3695:T24)  [unwired: 1 in]
                                n1262 = Bundle By Name(cluster=w3695, "lAO"=w3690, "lDO"=w3689, "Voltage step"=w3697, "Voltage triangle"=w3699, "file"=w3698) -> (w3696:T24)
                                n1263 = call "waveformparamsv2.vi"("Params in"=w3696, "command"="set") -> ()  [unwired: 1 out]
                                }
                                frame Enabled {
                                }
                                }
                                }
                                frame #2 {
                                n1264 = disable-structure shown="Disabled" {
                                frame Disabled {
                                n1265 = local read item#-1() -> (w3701)
                                n1266 = call "load waveforms.vi"("waveform"=w3701) -> ("# of points"=w3700:i32)
                                n1267 = local write "# of frames"(w3700) -> ()
                                }
                                frame Enabled {
                                }
                                }
                                }
                                }
                                }
                                }
                              }
                              frame #5 {
                                n1268 = call "2pparameters.vi"("command"="get") -> ("params out"=w3712:T12)  [unwired: 1 in]
                                n1269 = Unbundle By Name(w3712) -> ("refreshbuffer"=w3710:i32, "srate"=w3711:sgl)
                                n1270 = local read "wavdet"() -> (w3704:bool)
                                n1271 = case shown="True" w3704 {
                                tunnel: [w3719 w3720] -> w3703
                                frame False {
                                w3719 = 10123 items=["Finite Samples"=10178, "Continuous Samples"=10123, "Hardware Timed Single Point"=12522] ("sample mode")
                                }
                                frame True {
                                w3720 = 10123 items=["Finite Samples"=10178, "Continuous Samples"=10123, "Hardware Timed Single Point"=12522] ("sample mode")
                                }
                                }
                                n1272 = To Double Precision Float(number=w3711) -> (double precision float=w3714:dbl)
                                n1273 = To Double Precision Float(number=w3710) -> (double precision float=w3705:dbl)
                                n1274 = Divide(x=w3705, y=w3714) -> (x/y=w3718:dbl)
                                n1275 = Multiply(x=w3718, y=2.0) -> (x*y=w3715:dbl)
                                n1276 = Max & Min(x=w3715, y=10.0) -> (max(x,y)=w3706:dbl)  [unwired: 1 out]
                                n1277 = call "2pparameters.vi"("command"="get") -> ("params out"=w3709:T12)  [unwired: 1 in]
                                n1278 = Bundle By Name(cluster=w3709, "timeout"=w3706, "sample mode"=w3703) -> (w3707:T12)
                                n1279 = call "2pparameters.vi"("Params in"=w3707, "command"="set") -> ()  [unwired: 1 out]
                              }
                            }
                            n1280 = local write "data dir"(w3592) -> ()
                          }
                          frame #1 {
                            # "determine size of AI buffer still!!!"
                            # "counter needs a clock. rather than setting up a separate clock line\n (i have no more counters) I opt to always record an AI channel;\nin imaging i don't do this because the scanner provides a clock and the\nspeed needed to record at appreciable framerates makes it useful to limit the number of channels.\nin timetrace, the samplerate is unlikely to ever go over >10Ks/s so it matters less."
                            # "shutter line"
                            # "to patch and\nlaser (eventual aotf)"
                            n1281 = call "prepAO_tt_v2.vi"() -> ("Terminal Name with Device Prefix"=w3721:tag)  [unwired: 2 in]
                            n1282 = call "prepDO_tt.vi"() -> ()  [unwired: 2 in]
                            n1283 = call "prepAI_ttv2.vi"("triggersource"=w3721) -> ()  [unwired: 1 in, 1 out]
                            n1284 = call "prepCI_tt.vi"() -> ()  [unwired: 2 in]
                          }
                          frame #2 {
                            n1285 = local read "save\ndata"() -> (w3722:bool)
                            n1286 = case shown="True" w3722 {
                              tunnel: w3723 -> [_ w3727]
                              frame False {
                              }
                              frame True {
                                n1287 = local read "filename prefix"() -> (w3725:string)
                                n1288 = local read "data dir"() -> (w3726:path)
                                n1289 = call "preparebinaryfiles.vi"("filename prefix"=w3725, "data dir"=w3726, "timestamp"=w3727) -> ("full-filename"=w3724:string)  [unwired: 1 in]
                                n1290 = local write "full-filename"(w3724) -> ()
                              }
                            }
                          }
                          frame #3 {
                            n1291 = call "2pparameters.vi"("command"="get") -> ("params out"=w3729:T12)  [unwired: 1 in]
                            n1292 = Unbundle By Name(w3729) -> ("autoshutter"=w3730:bool)
                            n1293 = case shown="True" w3730 {
                              frame False {
                              }
                              frame True {
                                n1294 = call "shuttercontrol.vi"("command"="open") -> ()  [unwired: 1 in, 1 out]
                              }
                            }
                          }
                          frame #4 {
                            n1295 = flat-sequence {
                              frame #0 {
                                n1296 = call "runAI_img.vi"() -> ()  [unwired: 12 in]
                                n1297 = call "runCI.vi"() -> ()  [unwired: 12 in]
                                n1298 = call "runDO_img.vi"() -> ()  [unwired: 12 in]
                                n1299 = call "runAO_img.vi"() -> ()  [unwired: 12 in]
                              }
                              frame #1 {
                              }
                            }
                          }
                          frame #5 {
                            n1300 = while {
                              i -> [w3734]
                              stop <- w3732 stop-if-true
                              n1301 = local read "Stop"() -> (w3742:bool)
                              n1302 = local read "Exit"() -> (w3741:bool)
                              n1303 = Increment(x=w3734) -> (x+1=w3733:i32)
                              n1304 = local write "points recorded"(w3733) -> ()
                              n1305 = Or(x=w3742, y=w3741) -> (x .or. y?=w3740:bool)
                              n1306 = case shown="False" w3740 {
                                frame False {
                                n1307 = stacked-sequence {
                                frame #0 {
                                n1308 = call "collectCI_tt.vi"() -> ("size(s)"=w3749:i32)  [unwired: 3 in]
                                n1309 = local write "scol"(w3749) -> ()
                                n1310 = call "collectAI_tt_V2.vi"() -> ()  [unwired: 4 in]
                                }
                                frame #1 {
                                n1311 = local read "graph2list"() -> (w3754:u16)
                                n1312 = local read "graph1list"() -> (w3755:u16)
                                n1313 = To Unsigned Word Integer(number=w3754) -> (unsigned 16bit integer=w3757:u16)
                                n1314 = To Unsigned Word Integer(number=w3755) -> (unsigned 16bit integer=w3758:u16)
                                n1315 = local read "bin"() -> (w3762:dbl)
                                n1316 = call "dattotrace.vi"("graph2list"=w3757, "Current Average"=sgl 1.0, "graph1list"=w3758) -> ("trace2array out"=w3760:sgl[], "trace1array out"=w3759:sgl[])
                                n1317 = Array Size(array=w3760) -> (size(s)=w3763:i32)
                                n1318 = Divide(x=w3763, y=2) -> (x/y=w3765:dbl)
                                n1319 = Round To Nearest(number=w3765) -> (nearest integer value=w3767:dbl)
                                n1320 = script code="data=reshape(datain,[bin length(datain)./bin]);\ndataout=mean(data,1);"("bin"=w3762, "datain"=w3759) -> ("dataout"=w3761:dbl[])  [unwired: 1 in, 1 out]
                                n1321 = Array Size(array=w3761) -> (size(s)=w3772:i32)
                                n1322 = Delete From Array(array=w3760, length=w3767, index=0) -> (deleted portion=w3751:sgl[], array with subset deleted=w3750:sgl[])
                                n1323 = Divide(x=w3772, y=2) -> (x/y=w3770:dbl)
                                n1324 = Round To Nearest(number=w3770) -> (nearest integer value=w3768:dbl)
                                n1325 = Delete From Array(array=w3761, length=w3768, index=0) -> (deleted portion=w3752:dbl[], array with subset deleted=w3753:dbl[])
                                n1326 = local write "graph4"(w3750) -> ()
                                n1327 = local write "graph2"(w3753) -> ()
                                n1328 = local write "graph3"(w3751) -> ()
                                n1329 = local write "graph1"(w3752) -> ()
                                }
                                frame #2 {
                                n1330 = local read "save\ndata"() -> (w3773:bool)
                                n1331 = case shown="True" w3773 {
                                frame False {
                                }
                                frame True {
                                n1332 = call "savebinaryfiles.vi"() -> ()  [unwired: 1 in]
                                }
                                }
                                }
                                }
                                }
                                frame True {
                                }
                              }
                              n1333 = local read "continuous"() -> (w3737:bool)
                              n1334 = case shown="False" w3737 {
                                tunnel: w3733 -> [w3747 _]
                                tunnel: [w3746 FALSE] -> w3735
                                frame False {
                                n1335 = call "2pparameters.vi"("command"="get") -> ("params out"=w3744:T12)  [unwired: 1 in]
                                n1336 = Unbundle By Name(w3744) -> ("tt_cycles"=w3743:i32)
                                n1337 = Greater Or Equal?(x=w3747, y=w3743) -> (x >= y?=w3746:bool)
                                }
                                frame True {
                                }
                              }
                              n1338 = local read "Stop"() -> (w3739:bool)
                              n1339 = local read "Exit"() -> (w3738:bool)
                              n1340 = Or(x=w3739, y=w3738) -> (x .or. y?=w3736:bool)
                              n1341 = Or(x=w3736, y=w3735) -> (x .or. y?=w3732:bool)
                            }
                          }
                          frame #6 {
                            n1342 = call "stoperaseCI.vi"() -> ()  [unwired: 12 in]
                            n1343 = call "stoperaseDO_img.vi"() -> ()  [unwired: 12 in]
                            n1344 = call "stoperaseAO_img.vi"() -> ()  [unwired: 12 in]
                            n1345 = call "stoperaseAI_img.vi"() -> ()  [unwired: 12 in]
                          }
                          frame #7 {
                            w3776 = T23 2 items=["no dialog", "OK message", "continue or stop message", "OK message + warnings", "continue/stop + warnings"] ("type of dialog (OK msg:1)")
